vi "Distance to RPM.vi"(0 "Distance":dbl, 1 "Hoop":T1(ring)) -> (7 "Shooter RPM":dbl)   [LabVIEW 2011]
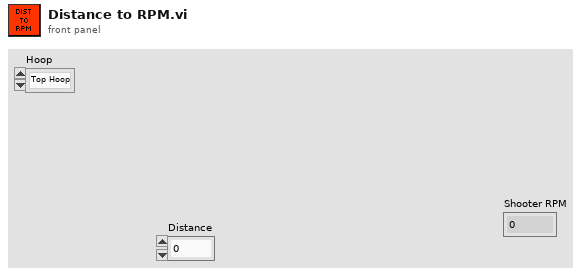
[diagram p1: front panel]
types:
  T1 = enum32{"Top Hoop", "Bottom Hoop", "Left Hoop", "Right Hoop"}
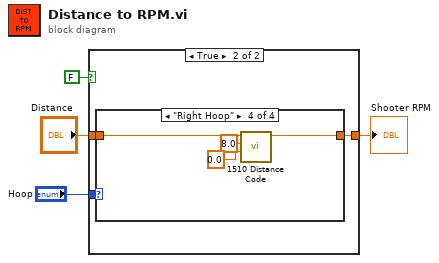
[diagram p0: block diagram]
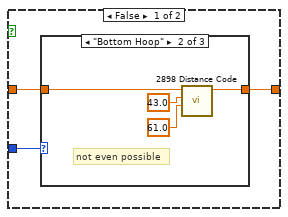
[diagram p2: hidden frame]
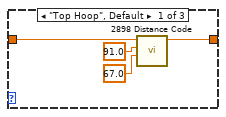
[diagram p3: hidden frame]
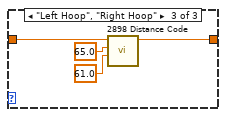
[diagram p4: hidden frame]
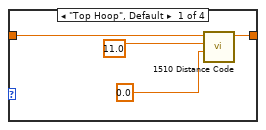
[diagram p5: hidden frame]
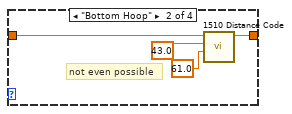
[diagram p6: hidden frame]
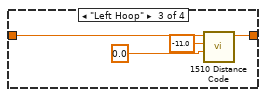
[diagram p7: hidden frame]
diagram:
  n1 = case shown="True" FALSE {
    tunnel: "Hoop" -> [w5 w22]
    tunnel: [w7 w21] -> w1
    tunnel: "Distance" -> [w6 w20]
    frame False {
      n2 = case shown="\"Bottom Hoop\"" w5 {
        tunnel: [w8 w14 w16] -> w7
        tunnel: w6 -> [w9 w15 w17]
        frame "Top Hoop", Default {
          n3 = call "2898 Distance Code.vi"("Cannon Height in Inches"=67.0, "Target Height in Inches"=91.0, "Distance to Shoot In Feet"=w9) -> ("Wheel RPM"=w8:dbl)  [unwired: 8 in]
        }
        frame "Bottom Hoop" {
          # "not even possible"
          n4 = call "2898 Distance Code.vi"("Cannon Height in Inches"=61.0, "Target Height in Inches"=43.0, "Distance to Shoot In Feet"=w15) -> ("Wheel RPM"=w14:dbl)  [unwired: 8 in]
        }
        frame "Left Hoop", "Right Hoop" {
          n5 = call "2898 Distance Code.vi"("Cannon Height in Inches"=61.0, "Target Height in Inches"=65.0, "Distance to Shoot In Feet"=w17) -> ("Wheel RPM"=w16:dbl)  [unwired: 8 in]
        }
      }
    }
    frame True {
      n6 = case shown="\"Right Hoop\"" w22 {
        tunnel: [w24 w30 w33 w36] -> w21
        tunnel: w20 -> [w25 w29 w34 w37]
        frame "Top Hoop", Default {
          n7 = call "1510 Distance Code.vi"("Cannon Height in Inches"=0.0, "Target Height in Inches"=11.0, "Distance to Shoot In Feet"=w25) -> ("Wheel RPM"=w24:dbl)  [unwired: 8 in]
        }
        frame "Bottom Hoop" {
          # "not even possible"
          n8 = call "1510 Distance Code.vi"("Cannon Height in Inches"=61.0, "Target Height in Inches"=43.0, "Distance to Shoot In Feet"=w29) -> ("Wheel RPM"=w30:dbl)  [unwired: 8 in]
        }
        frame "Left Hoop" {
          n9 = call "1510 Distance Code.vi"("Cannon Height in Inches"=0.0, "Target Height in Inches"=-11.0, "Distance to Shoot In Feet"=w34) -> ("Wheel RPM"=w33:dbl)  [unwired: 8 in]
        }
        frame "Right Hoop" {
          n10 = call "1510 Distance Code.vi"("Cannon Height in Inches"=0.0, "Target Height in Inches"=8.0, "Distance to Shoot In Feet"=w37) -> ("Wheel RPM"=w36:dbl)  [unwired: 8 in]
        }
      }
    }
  }
  "Shooter RPM" <- w1
